vi "Write HW ID.vi"(8 "error in (no error)":errorcluster, 10 "HW ID":dbl, 11 "Business Logic in":refnum<class "Business Logic.lvclass">) -> (0 "error out":errorcluster, 3 "Business Logic out":refnum<class "Business Logic.lvclass">)   [LabVIEW 2020, in "Business Logic.lvlib" / "Business Logic.lvclass"]
uses:
  Business Logic.lvclass
  Business Logic.lvclass/Business Logic.ctl
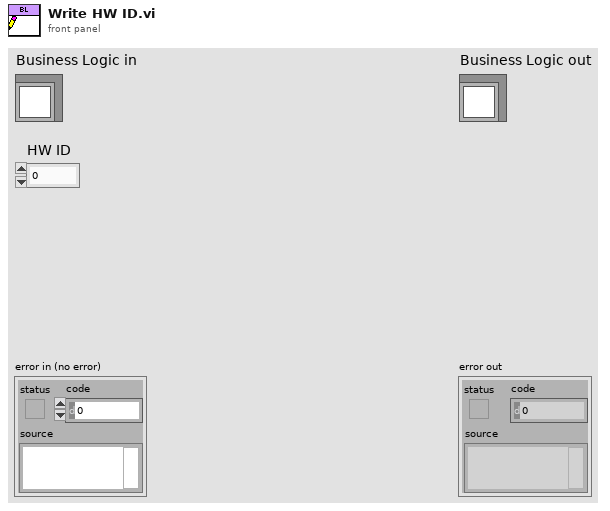
[diagram p1: front panel]
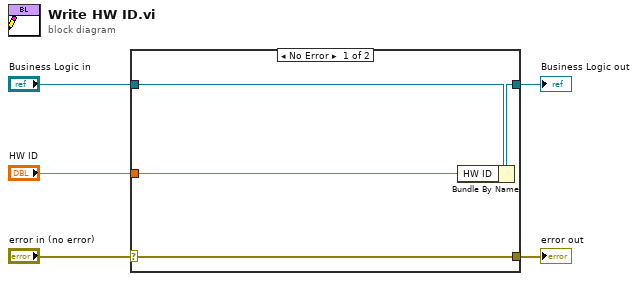
[diagram p0: block diagram]
diagram:
  n1 = case shown="No Error" "error in (no error)" {
    selector: "error in (no error)" -> [w9 w10]
    tunnel: [w9 w10] -> w4
    tunnel: [w7 w11] -> w2
    tunnel: "Business Logic in" -> [w8 w11]
    tunnel: "HW ID" -> [w6 _]
    frame No Error {
      n2 = Bundle By Name(cluster=w8, "HW ID"=w6) -> (w7:refnum<class "Business Logic.lvclass">)
    }
    frame Error {
    }
  }
  "error out" <- w4
  "Business Logic out" <- w2
